vi "Read Dependencies.vi"(8 "error in (no error)":errorcluster, 11 "SweepControl in":refnum<class "Sweep Control.lvclass">) -> (0 "error out":errorcluster, 2 "Transport":refnum<class "Transport.lvclass">, 3 "SweepControl out":refnum<class "Sweep Control.lvclass">)   [LabVIEW 2019, in "Sweep Control.lvclass"]
uses:
  Sweep Control.lvclass
  <userlib>/LevyLab/Transport/Transport/Transport.lvclass
  Sweep Control.lvclass/Sweep Control.ctl
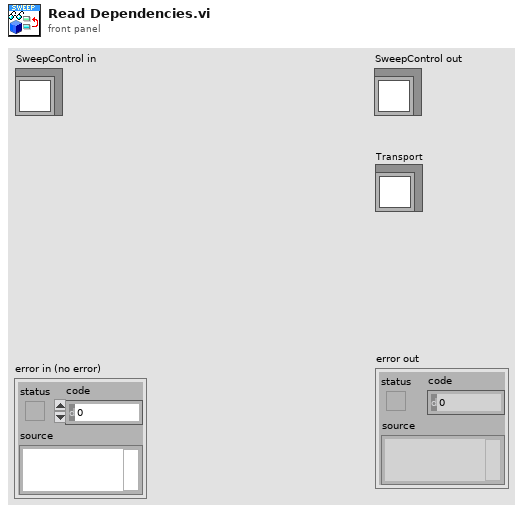
[diagram p1: front panel]
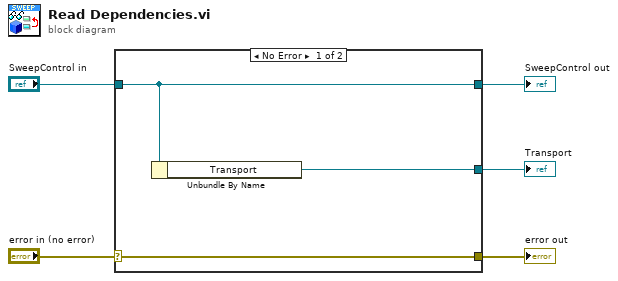
[diagram p0: block diagram]
diagram:
  n1 = case shown="No Error" "error in (no error)" {
    selector: "error in (no error)" -> [w8 w9]
    tunnel: [w8 w9] -> w4
    tunnel: [w7 w10] -> w2
    tunnel: "SweepControl in" -> [w7 w10]
    tunnel: [w6 _] -> w1
    frame No Error {
      n2 = Unbundle By Name(w7) -> ("Transport"=w6:refnum<class "Transport.lvclass">)
    }
    frame Error {
    }
  }
  "error out" <- w4
  "SweepControl out" <- w2
  "Transport" <- w1
